vi "Each Directive.vi"(4 "Template":string, 6 "Locals":refnum<class "Value Tree.lvclass">, 7 "Folder":path, 8 "error in (no error)":errorcluster, 9 "Value Name":string, 10 "Directive":string, 11 "BasicTemplater in":refnum<class "BasicTemplater.lvclass">) -> (0 "error out":errorcluster, 2 "Value":refnum<class "Value Tree.lvclass">, 3 "BasicTemplater out":refnum<class "BasicTemplater.lvclass">)   [LabVIEW 2020, in "HTTP Server.lvlib" / "BasicTemplater.lvclass"]
uses:
  BasicTemplater.lvclass
  Value Tree/Value Tree.lvclass
  Value Tree/Value Tree.lvclass/Value Tree.ctl
  BasicTemplater.lvclass/BasicTemplater.ctl
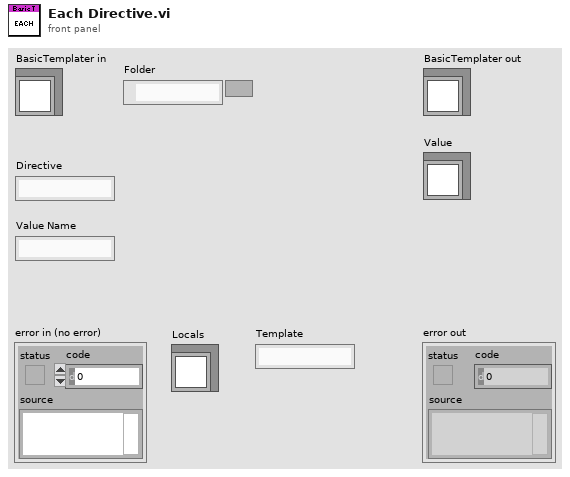
[diagram p1: front panel]
types:
  T1 = typedef "HTTP Server.lvlib/Value Tree.lvclass/Local Type.ctl" = enum16{"Scalar", "Object", "Array"}
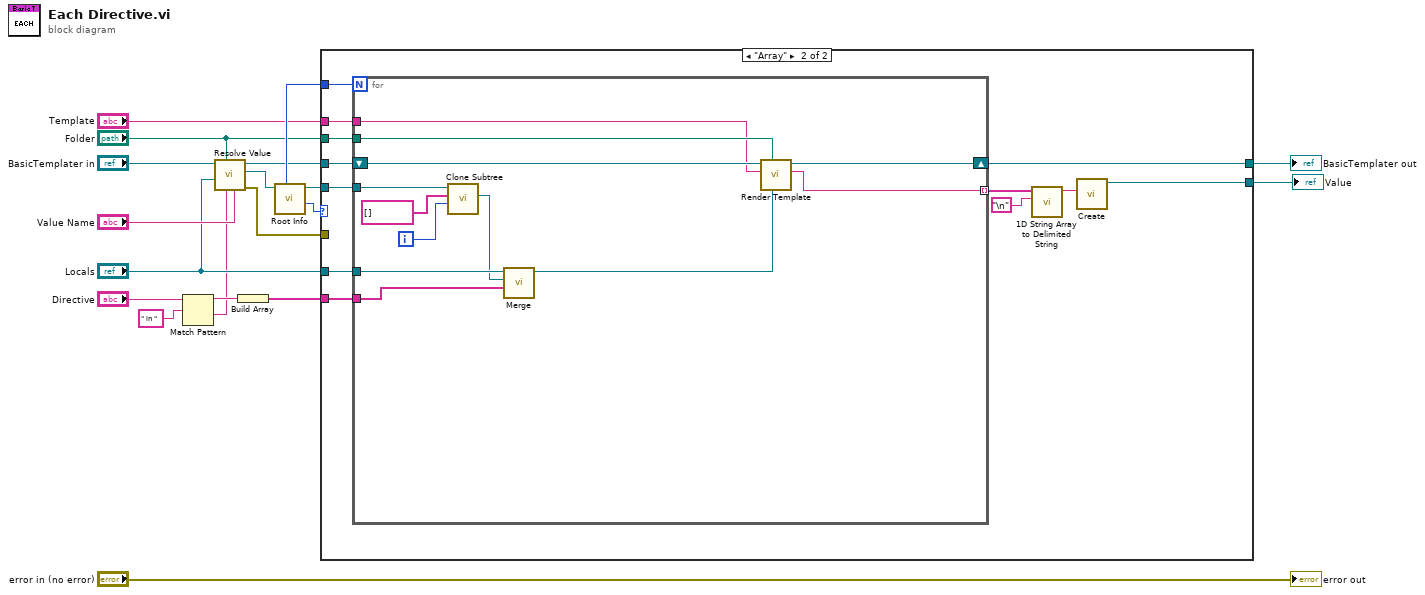
[diagram p0: block diagram]
diagram:
  n1 = Match Pattern(string="Directive", regular expression=" in ") -> (before substring=w3:string, after substring=w2:string)  [unwired: 1 in, 2 out]
  n2 = call "Resolve Value.vi"("Value Name"="Value Name", "Namespace"=w2, "Folder"="Folder", "Locals in"="Locals", "BasicTemplater in"="BasicTemplater in") -> ("error out"=w16:errorcluster, "Value"=w14:refnum<class "Value Tree.lvclass">, "BasicTemplater out"=w9:refnum<class "BasicTemplater.lvclass">)  [unwired: 4 in]
  n3 = Build Array(w3) -> (w10:string[])
  n4 = call "Root Info.vi"("Value Tree in"=w14) -> ("Type"=w13:T1, "Value Tree out"=w11:refnum<class "Value Tree.lvclass">, "Size"=w12:i32)  [unwired: 6 in, 2 out]
  n5 = case shown="\"Array\"" w13 {
    tunnel: w16 -> [_ _]
    tunnel: "Locals" -> [_ w32]
    tunnel: w12 -> [_ w31]
    tunnel: w11 -> [_ w30]
    tunnel: w10 -> [_ w29]
    tunnel: w9 -> [w20 w28]
    tunnel: [w20 w27] -> w8
    tunnel: "Folder" -> [_ w26]
    tunnel: [_ w22] -> w6
    tunnel: "Template" -> [_ w21]
    frame Default {
    }
    frame "Array" {
      n6 = for {
        N: w31 -> [_]
        tunnel: w32 -> [w41]
        tunnel: w30 -> [w44]
        tunnel: w29 -> [w40]
        shift-right: [w36] -> w27
        shift-left: w28 -> [w38]
        tunnel: w26 -> [w37]
        tunnel: [w35] -> w25 mode=indexing
        tunnel: w21 -> [w33]
        i -> [w43]
        n7 = call "Clone Subtree.vi"("Array Index (None)"=w43, "Hierarchy"=string[] [], "Value Tree in"=w44) -> ("Subtree"=w39:refnum<class "Value Tree.lvclass">)  [unwired: 6 in, 2 out]
        n8 = call "Merge.vi"("Destination"=w40, "Source Tree"=w39, "Value Tree in"=w41) -> ("Value Tree out"=w34:refnum<class "Value Tree.lvclass">)  [unwired: 7 in, 1 out]
        n9 = call-dynamic "Render Template.vi"("Locals (None)"=w34, "Folder"=w37, "Template"=w33, "BasicTemplater in"=w38) -> ("Output"=w35:string, "BasicTemplater out"=w36:refnum<class "BasicTemplater.lvclass">)  [unwired: 5 in, 1 out]
      }
      n10 = call <vilib>:"1D String Array to Delimited String.vi"("delimiter"="\n", "string array"=w25) -> ("delimited string"=w23:string)  [unwired: 9 in]
      n11 = call "Create.vi"("Value"=w23) -> ("Value Tree out"=w22:refnum<class "Value Tree.lvclass">)  [unwired: 10 in]
    }
  }
  "BasicTemplater out" <- w8
  "Value" <- w6
  "error out" <- "error in (no error)"
